vi "Initialize Configuration Attribute.vi"(6 "Access Scope (RO)":T1, 7 "Attribute.Config in":refnum<class "Attribute.Config.lvclass">) -> (2 "Config Changed Event":refnum<user-event>, 3 "Attribute.Config":refnum<class "Attribute.Config.lvclass">)   [LabVIEW 2013, in "Attribute.Config.lvclass"]
uses:
  Attribute.Config.lvclass
  AccessScope.ctl
  Definitions/def.SMO/Scope -- Enum.ctl
  Attribute/Attribute.lvclass/Attribute.ctl
  Attribute.Config.lvclass/Attribute.Config.ctl
  Attribute/Attribute.lvclass
  Definitions/def.SMO/def.SMO.lvclass
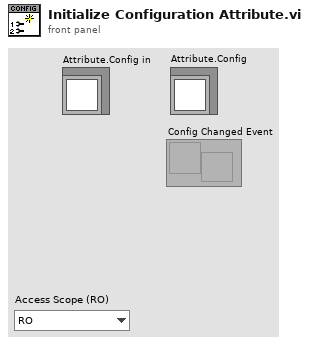
[diagram p1: front panel]
types:
  T1 = typedef "Attribute.Config.lvclass/AccessScope.ctl" = enum16{"RO", "RW"}
  T2 = typedef "def.SMO.lvclass/Scope -- Enum.ctl" = enum16{"Public", "Protected", "Private"}
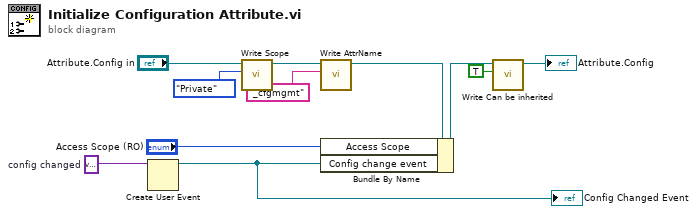
[diagram p0: block diagram]
diagram:
  w10 = variant  # config changed
  n1 = Create User Event(user event datatype=w10) -> (user event=w9:refnum<user-event>)  [unwired: 1 in, 1 out]
  "Config Changed Event" <- w9
  n2 = call "Write Scope.vi"("Scope"=Scope_--_Enum."Private", "Attribute in"="Attribute.Config in") -> ("Attribute out"=w6:refnum<class "Attribute.Config.lvclass">)  [unwired: 9 in]
  n3 = call "Write AttrName.vi"("Attribute Name"="_cfgmgmt", "Attribute in"=w6) -> ("Attribute out"=w2:refnum<class "Attribute.Config.lvclass">)  [unwired: 9 in]
  n4 = Bundle By Name(cluster=w2, "Access Scope"="Access Scope (RO)", "Config change event"=w9) -> (w8:refnum<class "Attribute.Config.lvclass">)
  n5 = call "Write Can be inherited.vi"("Can be inherited"=TRUE, "Attribute in"=w8) -> ("Attribute out"=→"Attribute.Config":refnum<class "Attribute.Config.lvclass">)  [unwired: 8 in, 1 out]
